vi "Convert to date-first Timestamp.vi"(4 "DTTM (Now)":timestamp) -> (1 "insertion string":string)   [LabVIEW 2022 SP3, in "hse-db-ado.lvlib" / "ADO-DB-Driver.lvlib"]
doc: "Convert timestamp to \"MM/DD/YYYY HH:MM:SS\"\n\n____\nHAMPEL SOFTWARE ENGINEERING v1.4.0 (2023-12-19 09:52)"
uses:
  ADO-DB-Driver.lvlib
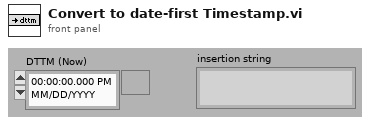
[diagram p1: front panel]
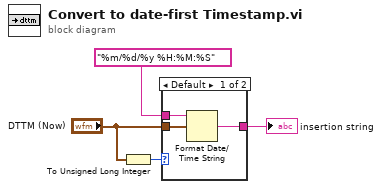
[diagram p0: block diagram]
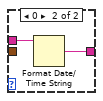
[diagram p2: hidden frame]
diagram:
  n1 = To Unsigned Long Integer(number="DTTM (Now)") -> (unsigned 32bit integer=w1:u32)
  n2 = case shown="Default" w1 {
    tunnel: "DTTM (Now)" -> [w7 _]
    tunnel: [w6 w9] -> w4
    tunnel: "%m/%d/%y %H:%M:%S" -> [w5 w8]
    frame Default {
      n3 = Format Date/Time String(time format string (%c)=w5, seconds (now)=w7) -> (date/time string=w6:string)  [unwired: 1 in]
    }
    frame 0 {
      n4 = Format Date/Time String(time format string (%c)=w8) -> (date/time string=w9:string)  [unwired: 2 in]
    }
  }
  "insertion string" <- w4
